vi "Set Strain.vi"(6 "Channel":i32=1 min=1 max=2, 8 "error in (no error)":errorcluster, 9 "Slew (V/s)":dbl, 10 "Strain (V)":dbl, 11 "Inst.RP100 in":refnum<class "Inst.RP100.lvclass">) -> (0 "error out":errorcluster, 3 "Inst.RP100 out":refnum<class "Inst.RP100.lvclass">)   [LabVIEW 2019, in "Inst.RP100.lvclass"]
doc: "Set the output <b>Strain</b> with <b>Slew</b> such that Channel 1 = -Channel 2. \n\n<b>Output Channel</b> is not used."
uses:
  Inst.RP100.lvclass
  C:/Program Files (x86)/National Instruments/LabVIEW 2019/user.lib/LevyLab/Instrument Framework/SMOs/Instrument/Instrument.lvclass
  Typedefs/SetStrain--Cluster.ctl
  Typedefs/Commands--Enum.ctl
  <userlib>/LevyLab/Instrument Framework/SMOs/Instrument/Instrument.lvclass/Instrument.ctl
  45516a56-4f23-4429-9a1b-5ca20d98b11a.vi
  45516a56-4f23-4429-9a1b-5ca20d98b11a.vi/cb49357b-e774-45c8-b665-8130b9809af8.vi
  45516a56-4f23-4429-9a1b-5ca20d98b11a.vi/cb49357b-e774-45c8-b665-8130b9809af8.vi/2a42711f-cebc-4b74-8952-eb30738ed5a0.vi
  <userlib>/LevyLab/Instrument Framework/SMOs/Instrument/API/Send and Receive.vi
  45516a56-4f23-4429-9a1b-5ca20d98b11a.vi/cb49357b-e774-45c8-b665-8130b9809af8.vi/f428709f-eee8-4382-92b6-f27fe5012243.vi
  <userlib>/LevyLab/Instrument Framework/SMOs/Instrument/Private/Get Client Type.vi
  45516a56-4f23-4429-9a1b-5ca20d98b11a.vi/cb49357b-e774-45c8-b665-8130b9809af8.vi/2a42711f-cebc-4b74-8952-eb30738ed5a0.vi/77d53d02-9725-4bd6-bd0f-771020def231.vi
  45516a56-4f23-4429-9a1b-5ca20d98b11a.vi/cb49357b-e774-45c8-b665-8130b9809af8.vi/2a42711f-cebc-4b74-8952-eb30738ed5a0.vi/4d63478f-a6f7-442b-825a-41dd3b894dac.vi
  45516a56-4f23-4429-9a1b-5ca20d98b11a.vi/cb49357b-e774-45c8-b665-8130b9809af8.vi/f428709f-eee8-4382-92b6-f27fe5012243.vi/e6df3129-a235-4887-8486-55c66d7b72a2.vi
  45516a56-4f23-4429-9a1b-5ca20d98b11a.vi/cb49357b-e774-45c8-b665-8130b9809af8.vi/f428709f-eee8-4382-92b6-f27fe5012243.vi/25127783-e326-4440-91e5-e585362da746.vi
  45516a56-4f23-4429-9a1b-5ca20d98b11a.vi/cb49357b-e774-45c8-b665-8130b9809af8.vi/f428709f-eee8-4382-92b6-f27fe5012243.vi/e6df3129-a235-4887-8486-55c66d7b72a2.vi/eea4b55a-4bc5-4a74-b0b1-8ba6b05779b2.vi
  45516a56-4f23-4429-9a1b-5ca20d98b11a.vi/cb49357b-e774-45c8-b665-8130b9809af8.vi/f428709f-eee8-4382-92b6-f27fe5012243.vi/e6df3129-a235-4887-8486-55c66d7b72a2.vi/654e776d-6ed7-4fba-b1a0-0aa8a4eb2eb2.vi
  <userlib>/LevyLab/Instrument Framework/SMOs/Instrument/Private/Get RC Connection Status.vi
  <userlib>/LevyLab/Instrument Framework/SMOs/Instrument/API/Enum to String.vi
  <userlib>/LevyLab/Instrument Framework/SMOs/RemoteControl/API/Send and Receive.vi
  <vilib>/Utility/Data Type/Get Type Information.vi
  <vilib>/JDP Science/JSONtext/JSON text to Variant.vi
  <userlib>/LevyLab/Instrument Framework/SMOs/Instrument/API/Instrument.GetPublicEvents.vi
  <vilib>/JDP Science/JSONtext/Variant to JSON Text.vi
  <vilib>/National Instruments/GUID Generator/Guid Generator.vi
  <userlib>/LevyLab/Instrument Framework/SMOs/Instrument/API/Instrument.MessageToProcess.vi
  <userlib>/LevyLab/Instrument Framework/SMOs/Instrument/Private/Instrument.MessageFromProcess.EventStructure.vi
  <vilib>/JDP Science/JSONtext/LVClass Serializer/JSONtext LVClass Serializer.lvclass
panel:
  # "legacy (not used)"
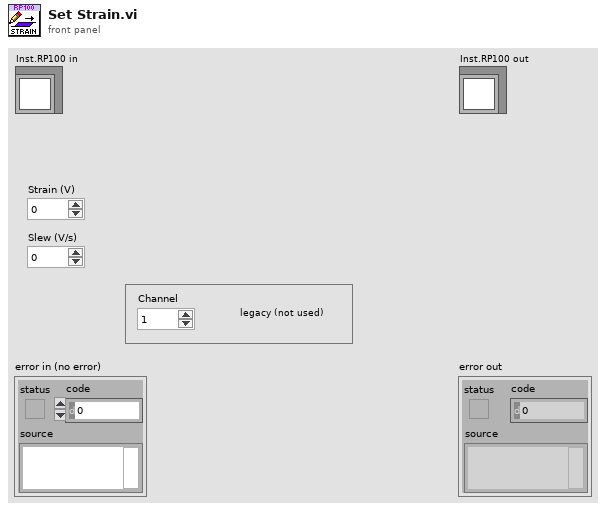
[diagram p1: front panel]
types:
  T1 = typedef "Inst.RP100.lvclass/Commands--Enum.ctl" = enum16{"setState", "setStrain", "getStrain", "setLevel", "getLevel"}
  T2 = typedef "Inst.RP100.lvclass/SetStrain--Cluster.ctl" = cluster{"Strain (V)":dbl, "Slew (V/s)":dbl}
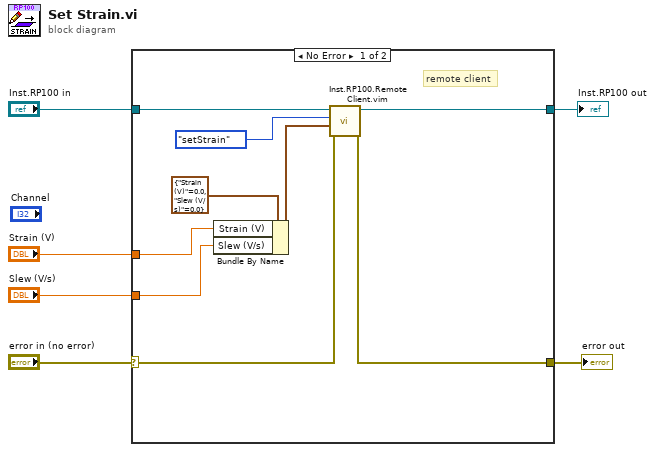
[diagram p0: block diagram]
diagram:
  n1 = case shown="No Error" "error in (no error)" {
    selector: "error in (no error)" -> [w8 w17]
    tunnel: [w7 w17] -> w5
    tunnel: "Strain (V)" -> [w12 _]
    tunnel: "Inst.RP100 in" -> [w15 w16]
    tunnel: [w14 w16] -> w2
    tunnel: "Slew (V/s)" -> [w11 _]
    frame No Error {
      # "remote client"
      n2 = Bundle By Name(cluster=T2 {"Strain (V)"=0.0, "Slew (V/s)"=0.0} ("setStrain"), "Strain (V)"=w12, "Slew (V/s)"=w11) -> (w9:T2)
      n3 = call "Inst.RP100.Remote Client.vim"("error in (no error)"=w8, "params"=w9, "Commands"=Commands--Enum."setStrain", "Inst.RP100 in"=w15) -> ("error out"=w7:errorcluster, "Inst.RP100 out"=w14:refnum<class "Inst.RP100.lvclass">)  [unwired: 5 in, 1 out]
    }
    frame Error {
    }
  }
  "error out" <- w5
  "Inst.RP100 out" <- w2
